vi "Read Subroutine Name.vi"(11 "Subroutine Dialog in":refnum<class "Subroutine Dialog.lvclass">) -> (2 "Name":string, 3 "Subroutine Dialog out":refnum<class "Subroutine Dialog.lvclass">)   [LabVIEW 2017, in "Subroutine Dialog.lvclass"]
uses:
  <vilib>/gpm_packages/@cs/Test-executive-builder/Source/Test Executive Builder Dialogs/Edit Subroutine Dialog/Subroutine Dialog.lvclass
  <vilib>/gpm_packages/@cs/Test-executive-builder/Source/Test Executive Builder Dialogs/Edit Subroutine Dialog/Subroutine Dialog.lvclass/Subroutine Dialog.ctl
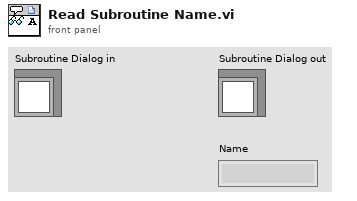
[diagram p1: front panel]
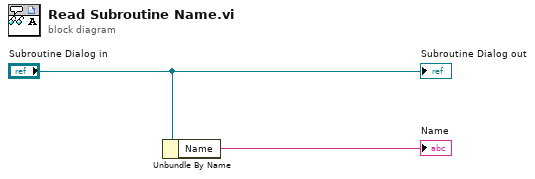
[diagram p0: block diagram]
diagram:
  n1 = Unbundle By Name("Subroutine Dialog in") -> ("Name"=→"Name":string)
  "Subroutine Dialog out" <- "Subroutine Dialog in"
